vi "FeedbackDecode_UpdateEncodeClust.vi"(2 "EncodeClustIn":T1={"ParamsTable"=[], "Sel"=[], "Stim"=FALSE, "StimMode"=enum."Off", "StimStep"=[enum."1uA", enum."1uA", enum."Off"], "Jitter"=FALSE, "Pulse"=FALSE, "BFreq"=0.0, "BAmp"=0.0, "UEAArray"=[], "AdjClust"={"Add"=FALSE, "Sub"=FALSE, "Val"=[1.0, 100.0, 0.2, 500.0, 0.0], "B"=[FALSE, FALSE, FALSE, FALSE, FALSE], "Inc+"=["x+1", "x+10", "x+0.1", "x+10", "x+10"], "Set"=FALSE, "LoadTable"=FALSE, "SaveTable"=FALSE, "ClearTable"=FALSE, "DeleteSel"=FALSE, "Inc-"=["x-1", "x-10", "x-0.1", "x-10", "x-10"]}, "PresetTable"=[], "SelPreset"=[], "SortClust"={"Region"=FALSE, "Receptor"=FALSE, "Electrode"=FALSE, "Min Amp"=FALSE, "Max Amp"=FALSE, "Min Freq"=FALSE, "Max Freq"=FALSE, "Duration"=FALSE}, "SelSort"={"Sel"=FALSE}, "PresetClust"={"Load"=FALSE, "Clear"=FALSE, "Save"=FALSE, "Del"=FALSE}, "RespClust"={"RespType"=enum."Sensor Map", "OpenResp"=FALSE}, "AmpLimit"=0.0, "FreqLimit"=0.0, "DurLimit"=0.0, "Wait Period"=0.0, "Train Period"=0.0, "ManualType"=enum."Max"} {"Train Period" min=0.0 max=100.0 step=0.1; "Wait Period" min=0.0 max=100.0 step=0.1; "DurLimit" min=0.0 max=1.0 step=0.01; "FreqLimit" min=0.0 max=500.0 step=1.0; "AmpLimit" min=0.0 max=100.0 step=1.0; "BAmp" min=0.0 max=100.0 step=1.0; "BFreq" min=0.0 max=100.0 step=1.0}, 3 "EvntStrIn":string) -> (0 "EncodeClustOut":T1={"ParamsTable"=[], "Sel"=[], "Stim"=FALSE, "StimMode"=enum."Off", "StimStep"=[enum."1uA", enum."1uA", enum."Off"], "Jitter"=FALSE, "Pulse"=FALSE, "BFreq"=0.0, "BAmp"=0.0, "UEAArray"=[], "AdjClust"={"Add"=FALSE, "Sub"=FALSE, "Val"=[1.0, 100.0, 0.2, 500.0, 0.0], "B"=[FALSE, FALSE, FALSE, FALSE, FALSE], "Inc+"=["x+1", "x+10", "x+0.1", "x+10", "x+10"], "Set"=FALSE, "LoadTable"=FALSE, "SaveTable"=FALSE, "ClearTable"=FALSE, "DeleteSel"=FALSE, "Inc-"=["x-1", "x-10", "x-0.1", "x-10", "x-10"]}, "PresetTable"=[], "SelPreset"=[], "SortClust"={"Region"=FALSE, "Receptor"=FALSE, "Electrode"=FALSE, "Min Amp"=FALSE, "Max Amp"=FALSE, "Min Freq"=FALSE, "Max Freq"=FALSE, "Duration"=FALSE}, "SelSort"={"Sel"=FALSE}, "PresetClust"={"Load"=FALSE, "Clear"=FALSE, "Save"=FALSE, "Del"=FALSE}, "RespClust"={"RespType"=enum."Sensor Map", "OpenResp"=FALSE}, "AmpLimit"=0.0, "FreqLimit"=0.0, "DurLimit"=0.0, "Wait Period"=0.0, "Train Period"=0.0, "ManualType"=enum."Max"} {"Train Period" min=0.0 max=100.0 step=0.1; "Wait Period" min=0.0 max=100.0 step=0.1; "DurLimit" min=0.0 max=1.0 step=0.01; "FreqLimit" min=0.0 max=500.0 step=1.0; "AmpLimit" min=0.0 max=100.0 step=1.0; "BAmp" min=0.0 max=100.0 step=1.0; "BFreq" min=0.0 max=100.0 step=1.0})   [LabVIEW 2020]
uses:
  FeedbackDecode_EncodeClust.ctl
  <vilib>/regexp/Match Regular Expression.xnode
panel:
  # "Value"
  # "Inc-"
  # "Inc+"
  # "Min Amp"
  # "Max Amp"
  # "Min Freq"
  # "Max Freq"
  # "Duration"
  # "Value"
  # "Inc-"
  # "Inc+"
  # "Min Amp"
  # "Max Amp"
  # "Min Freq"
  # "Max Freq"
  # "Duration"
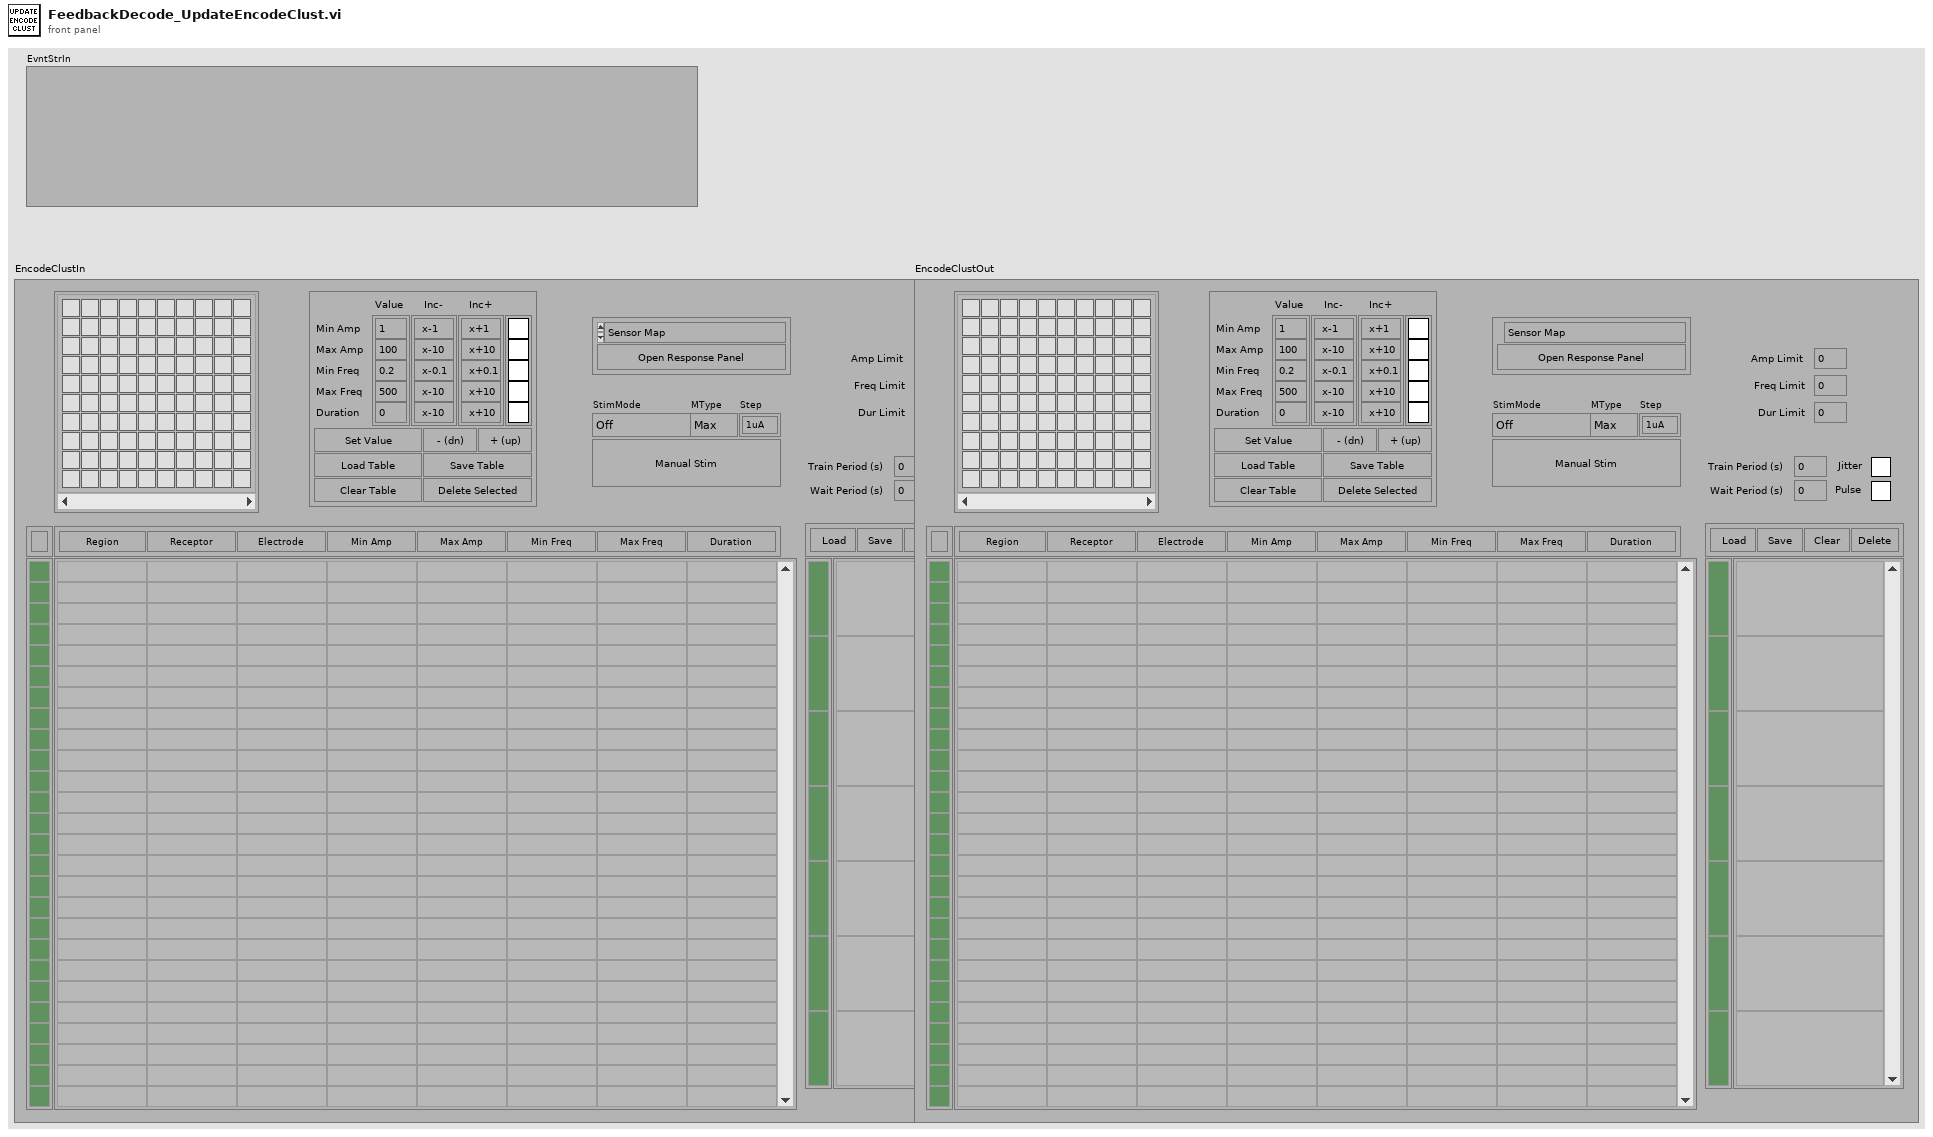
[diagram p1: front panel]
types:
  T1 = typedef "FeedbackDecode_EncodeClust.ctl" = cluster{"ParamsTable":string[][], "Sel":bool[], "Stim":bool, "StimMode":enum16{"Off", "Manual", "MSMS", "VRE", "3DHand", "DEKA", "Analog(DEKA)"}, "StimStep":enum16{"Off", "1uA", "2uA", "5uA", "10uA", "20uA", "30uA"}[], "Jitter":bool, "Pulse":bool, "BFreq":dbl, "BAmp":dbl, "UEAArray":cluster{"Boolean 1":bool, "Boolean 2":bool, "Boolean 3":bool, "Boolean 4":bool, "Boolean 5":bool, "Boolean 6":bool, "Boolean 7":bool, "Boolean 8":bool, "Boolean 9":bool, "Boolean 10":bool, "Boolean 11":bool, "Boolean 12":bool, "Boolean 13":bool, "Boolean 14":bool, "Boolean 15":bool, "Boolean 16":bool, "Boolean 17":bool, "Boolean 18":bool, "Boolean 19":bool, "Boolean 20":bool, "Boolean 21":bool, "Boolean 22":bool, "Boolean 23":bool, "Boolean 24":bool, "Boolean 25":bool, "Boolean 26":bool, "Boolean 27":bool, "Boolean 28":bool, "Boolean 29":bool, "Boolean 30":bool, "Boolean 31":bool, "Boolean 32":bool, "Boolean 33":bool, "Boolean 34":bool, "Boolean 35":bool, "Boolean 36":bool, "Boolean 37":bool, "Boolean 38":bool, "Boolean 39":bool, "Boolean 40":bool, "Boolean 41":bool, "Boolean 42":bool, "Boolean 43":bool, "Boolean 44":bool, "Boolean 45":bool, "Boolean 46":bool, "Boolean 47":bool, "Boolean 48":bool, "Boolean 49":bool, "Boolean 50":bool, "Boolean 51":bool, "Boolean 52":bool, "Boolean 53":bool, "Boolean 54":bool, "Boolean 55":bool, "Boolean 56":bool, "Boolean 57":bool, "Boolean 58":bool, "Boolean 59":bool, "Boolean 60":bool, "Boolean 61":bool, "Boolean 62":bool, "Boolean 63":bool, "Boolean 64":bool, "Boolean 65":bool, "Boolean 66":bool, "Boolean 67":bool, "Boolean 68":bool, "Boolean 69":bool, "Boolean 70":bool, "Boolean 71":bool, "Boolean 72":bool, "Boolean 73":bool, "Boolean 74":bool, "Boolean 75":bool, "Boolean 76":bool, "Boolean 77":bool, "Boolean 78":bool, "Boolean 79":bool, "Boolean 80":bool, "Boolean 81":bool, "Boolean 82":bool, "Boolean 83":bool, "Boolean 84":bool, "Boolean 85":bool, "Boolean 86":bool, "Boolean 87":bool, "Boolean 88":bool, "Boolean 89":bool, "Boolean 90":bool, "Boolean 91":bool, "Boolean 92":bool, "Boolean 93":bool, "Boolean 94":bool, "Boolean 95":bool, "Boolean 96":bool, "Boolean 97":bool, "Boolean 98":bool, "Boolean 99":bool, "Boolean 100":bool}[], "AdjClust":cluster{"Add":bool, "Sub":bool, "Val":dbl[], "B":bool[], "Inc+":string[], "Set":bool, "LoadTable":bool, "SaveTable":bool, "ClearTable":bool, "DeleteSel":bool, "Inc-":string[]}, "PresetTable":string[][], "SelPreset":bool[], "SortClust":cluster{"Region":bool, "Receptor":bool, "Electrode":bool, "Min Amp":bool, "Max Amp":bool, "Min Freq":bool, "Max Freq":bool, "Duration":bool}, "SelSort":cluster{"Sel":bool}, "PresetClust":cluster{"Load":bool, "Clear":bool, "Save":bool, "Del":bool}, "RespClust":cluster{"RespType":enum16{"Sensor Map", "Full Map"}, "OpenResp":bool}, "AmpLimit":dbl, "FreqLimit":dbl, "DurLimit":dbl, "Wait Period":dbl, "Train Period":dbl, "ManualType":enum16{"Max", "Min"}}
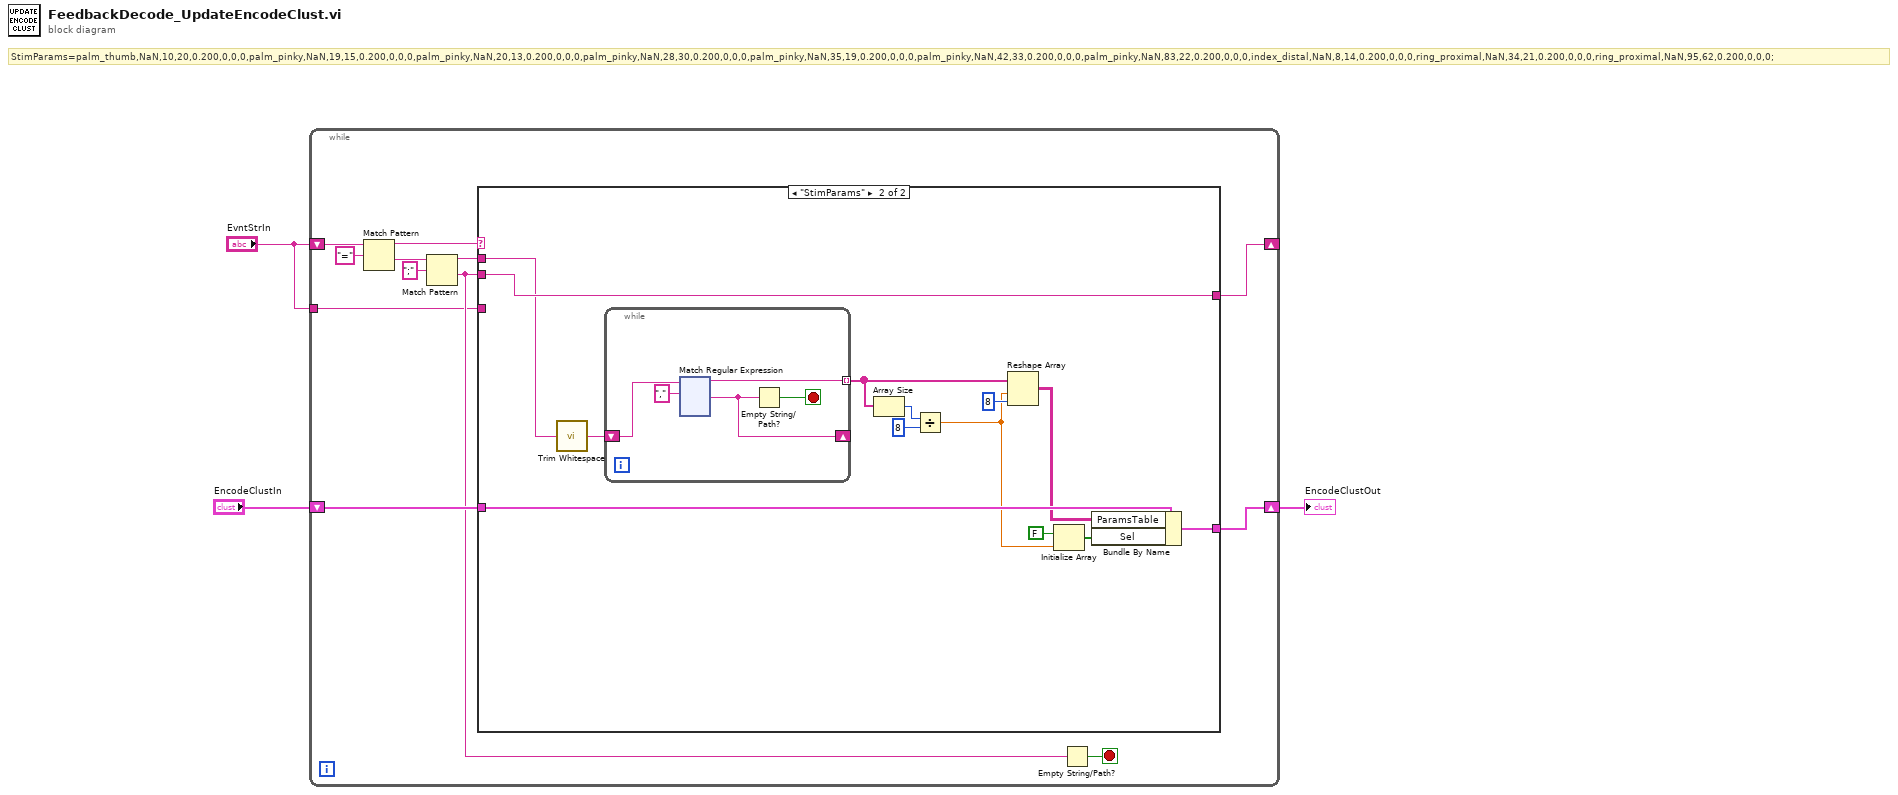
[diagram p0: block diagram]
diagram:
  # "StimParams=palm_thumb,NaN,10,20,0.200,0,0,0,palm_pinky,NaN,19,15,0.200,0,0,0,palm_pinky,NaN,20,13,0.200,0,0,0,palm_pinky,NaN,28,30,0.200,0,0,0,palm_pinky,NaN,35,19,0.200,0,0,0,palm_pinky,NaN,42,33,0.200,0,0,0,palm_pinky,NaN,83,22,0.200,0,0,0,index_distal,NaN,8,14,0.200,0,0,0,ring_proximal,NaN,34,21,0.200,0,0,0,ring_proximal,NaN,95,62,0.200,0,0,0;"
  n1 = while {
    shift-right: [w11] -> w2
    shift-left: "EncodeClustIn" -> [w12]
    shift-right: [w9] -> _
    shift-left: "EvntStrIn" -> [w15]
    tunnel: "EvntStrIn" -> [w4]
    stop <- w10 stop-if-true
    n2 = Match Pattern(string=w15, regular expression="=") -> (before substring=w13:string, after substring=w7:string)  [unwired: 1 in, 2 out]
    n3 = Match Pattern(string=w7, regular expression=";") -> (before substring=w6:string, after substring=w5:string)  [unwired: 1 in, 2 out]
    n4 = case shown="\"StimParams\"" w13 {
      tunnel: w12 -> [w16 w30]
      tunnel: [w16 w29] -> w11
      tunnel: [w17 w28] -> w9
      tunnel: w6 -> [_ w27]
      tunnel: w5 -> [w17 w28]
      tunnel: w4 -> [_ _]
      frame "", Default {
      }
      frame "StimParams" {
        n5 = call <vilib>:"Trim Whitespace.vi"("string"=w27) -> ("trimmed string"=w26:string)  [unwired: 1 in]
        n6 = while {
          shift-right: [w32] -> _
          shift-left: w26 -> [w34]
          tunnel: [w31] -> w23 mode=indexing
          stop <- w33 stop-if-true
          n7 = xnode "Match Regular Expression"("input string"=w34, "regular expression"=",") -> ("before match"=w31:string, "after match"=w32:string)  [unwired: 4 in, 3 out]
          n8 = Empty String/Path?(string/path=w32) -> (empty?=w33:bool)
        }
        n9 = Array Size(array=w23) -> (size(s)=w22:i32)
        n10 = Divide(x=w22, y=8) -> (x/y=w19:dbl)
        n11 = Reshape Array(w23, w19, 8 ("dimension size")) -> (w24:string[][])
        n12 = Initialize Array(FALSE, w19) -> (w18:bool[])
        n13 = Bundle By Name(cluster=w30, "ParamsTable"=w24, "Sel"=w18) -> (w29:T1)
      }
    }
    n14 = Empty String/Path?(string/path=w5) -> (empty?=w10:bool)
  }
  "EncodeClustOut" <- w2
